vi "h5_init_2D_config.vi"(7 "scan_config":T1={"v0 name"="radiant (nm)", "v0 num"=808, "v1 name"="none", "v1 num"=808, "scan_values"=[], "num rows"=808, "measurement"=0, "v0_config"={"hardware"=enum."radiant (nm)", "options"="", "repeats"=4, "loops"=1, "VISA"="COM9", "override_VISA"=TRUE}, "v1_config"={"hardware"=enum."radiant (nm)", "options"="", "repeats"=4, "loops"=1, "VISA"="COM9", "override_VISA"=TRUE}, "scope_config"={"VISA"="lecroy", "channels"=[enum."Channel 1"], "timeout (ms)"=100000, "max_points"=2500, "averages"=50, "noise filter"=enum."None"}} {"scope_config"."averages" min=1; "scope_config"."max_points" items=["50"=50, "100"=100, "250"=250, "500"=500, "1000"=1000, "2500"=2500, "5K"=5000, "10K"=10000, "25K"=25000, "50K"=50000, "100K"=100000, "250K"=250000, "500K"=500000, "1M"=1000000, "2M"=2000000, "2.5M"=2500000, "5M"=5000000, "10M"=10000000, "25M"=25000000, "50M"=50000000, "100M"=100000000]; "v1_config"."loops" min=1; "v1_config"."repeats" min=1; "v0_config"."loops" min=1; "v0_config"."repeats" min=1}) -> (15 "error out":errorcluster)   [LabVIEW 2017, in "tools.lvlib"]
uses:
  tools.lvlib
  <vilib>/UPVI/lvhdf5/attribute.llb/Simple H5Awrite.xnode
  <vilib>/UPVI/lvhdf5/attribute.llb/LVH5A Operation.ctl
  <vilib>/UPVI/lvhdf5/library.llb/HDF5 Ref.ctl
  <vilib>/UPVI/lvhdf5/attribute.llb/Simple H5Awrite (Variant).vi
  <vilib>/UPVI/lvhdf5/attribute.llb/Cluster to Attribute Array.xnode
  <vilib>/Utility/VariantDataType/GetClusterInfo.vi
  <vilib>/Utility/VariantDataType/VariantType.lvlib
  <vilib>/Utility/VariantDataType/GetTypeInfo.vi
  ctrl/var_list.ctl
  core/var_config.ctl
  hardware/lecroy/scope_config.ctl
  hardware/lecroy/lecroy.lvlib
  core/scan_config.ctl
panel:
  in  "scan_config 2":T1={"v0 name"="radiant (nm)", "v0 num"=808, "v1 name"="none", "v1 num"=808, "scan_values"=[], "num rows"=808, "measurement"=0, "v0_config"={"hardware"=enum."radiant (nm)", "options"="", "repeats"=4, "loops"=1, "VISA"="COM9", "override_VISA"=TRUE}, "v1_config"={"hardware"=enum."radiant (nm)", "options"="", "repeats"=4, "loops"=1, "VISA"="COM9", "override_VISA"=TRUE}, "scope_config"={"VISA"="lecroy", "channels"=[enum."Channel 1"], "timeout (ms)"=100000, "max_points"=2500, "averages"=50, "noise filter"=enum."None"}} {"scope_config"."averages" min=1; "scope_config"."max_points" items=["50"=50, "100"=100, "250"=250, "500"=500, "1000"=1000, "2500"=2500, "5K"=5000, "10K"=10000, "25K"=25000, "50K"=50000, "100K"=100000, "250K"=250000, "500K"=500000, "1M"=1000000, "2M"=2000000, "2.5M"=2500000, "5M"=5000000, "10M"=10000000, "25M"=25000000, "50M"=50000000, "100M"=100000000]; "v1_config"."loops" min=1; "v1_config"."repeats" min=1; "v0_config"."loops" min=1; "v0_config"."repeats" min=1}
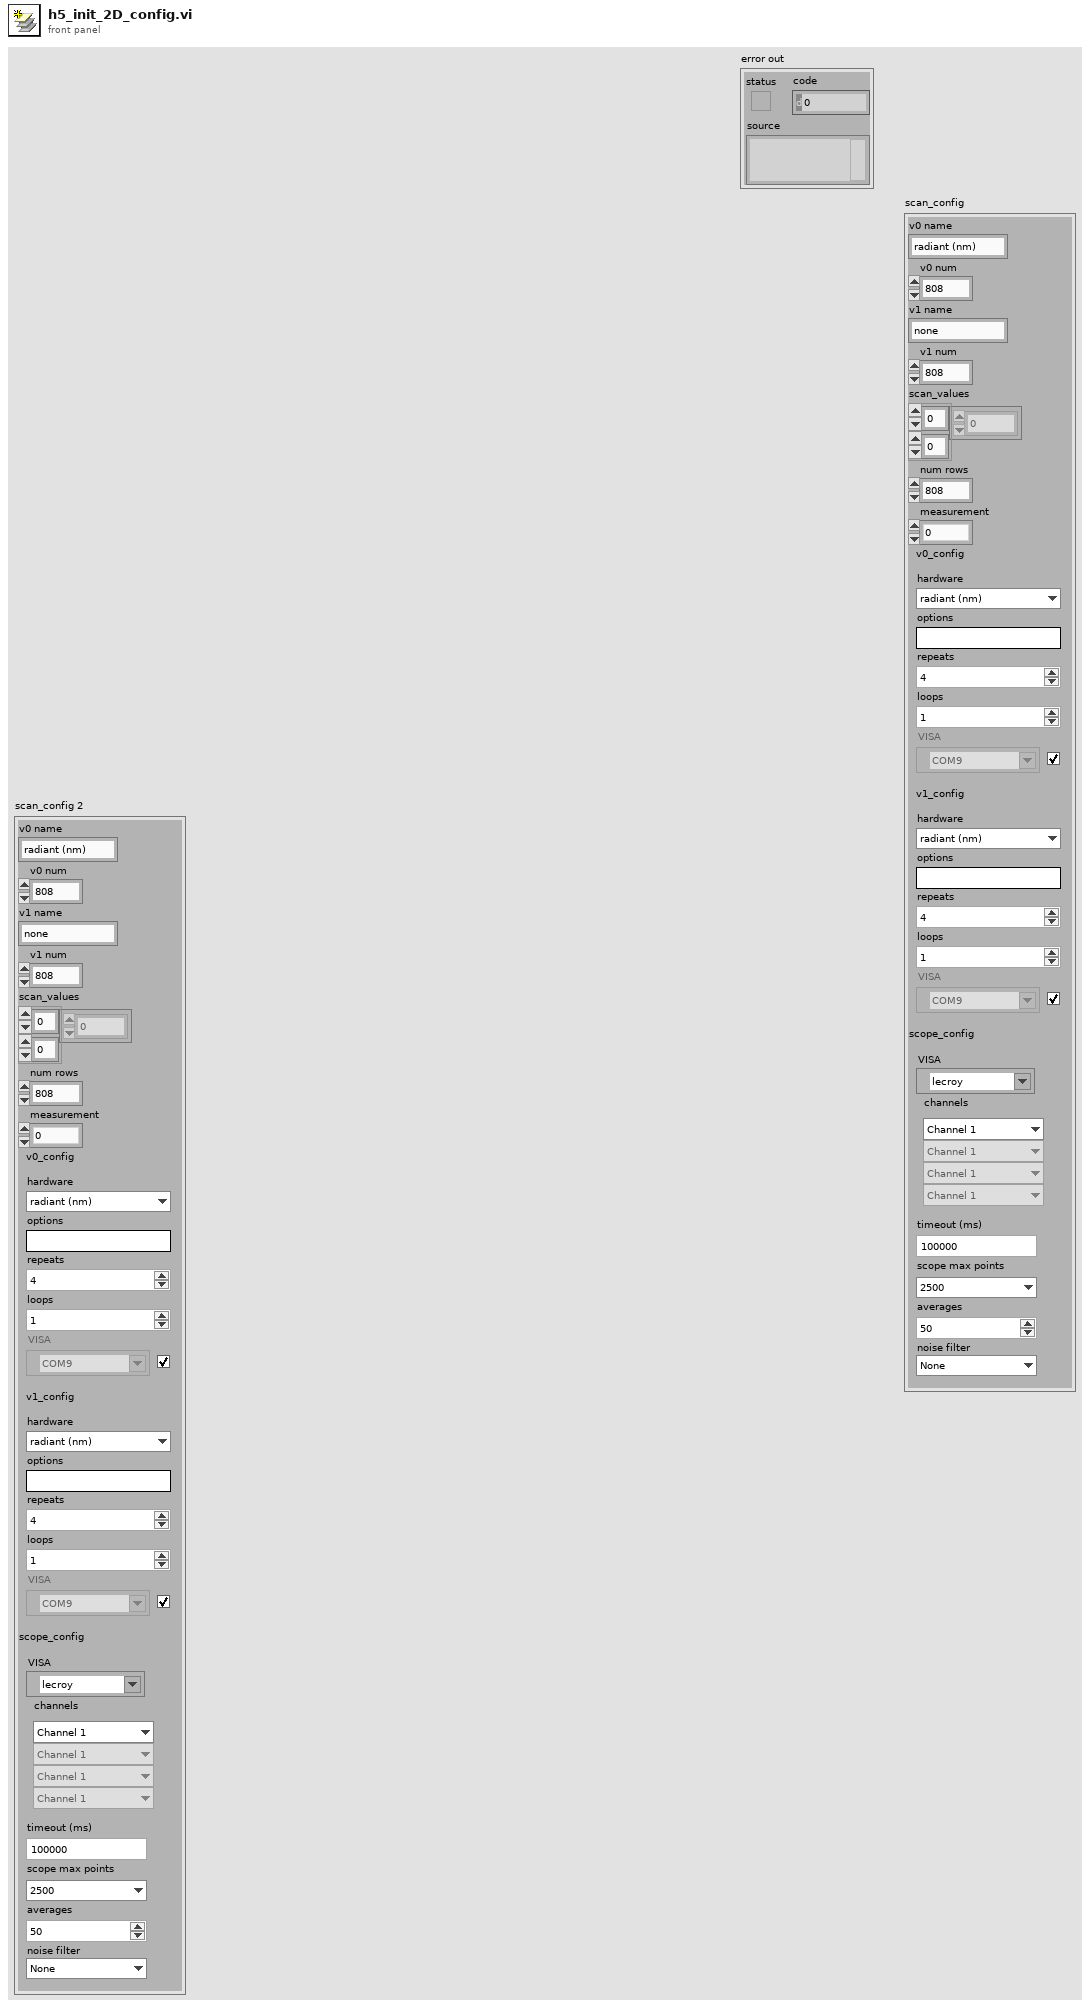
[diagram p1: front panel]
types:
  T1 = typedef "tools.lvlib/scan_config.ctl" = cluster{"v0 name":string, "v0 num":i32, "v1 name":string, "v1 num":i32, "scan_values":dbl[][], "num rows":i32, "measurement":i32, "v0_config":T2, "v1_config":T2, "scope_config":T4}
  T2 = typedef "tools.lvlib/var_config.ctl" = cluster{"hardware":T3, "options":string, "repeats":i32, "loops":i32, "VISA":refnum<visa-resource-name>, "override_VISA":bool}
  T3 = typedef "var_list.ctl" = enum16{"none", "AO voltage (V)", "delay (s)", "generic", "microwaves (GHz)", "radiant (nm)", "radiant thg (nm)", "sirah (nm)", "sirah_shg (nm)", "tenma voltage (V)", "wait (s)", "wf_freq (Hz)", "wf_amp (V)", "wf_amp_multi (V)", "wf_offset (V)", "wf_low_level (V)", "wf_high_level (V)", "wf_period (s)", "wf_pulse_width (s)", "wf_sample_rate (Sa/s)", "wf_multi_amp", "wf_multi_freq", "wf_arb_4chan", "WS7 setpoint (nm)"}
  T4 = typedef "lecroy.lvlib/scope_config.ctl" = cluster{"VISA":refnum<visa-resource-name>, "channels":enum16{"Channel 1", "Channel 2", "Channel 3", "Channel 4"}[], "timeout (ms)":u32, "max_points":i32, "averages":i32, "noise filter":enum16{"None", "+0.5 bit", "+1 bit", "+1.5 bits", "+2 bits", "+2.5 bits", "+3 bits"}}
  T5 = cluster{"num rows":i32, "v0_config":T2, "v1_config":T2, "scope_config":T4}
  T6 = typedef "HDF5 Ref.ctl" = refnum<k1>
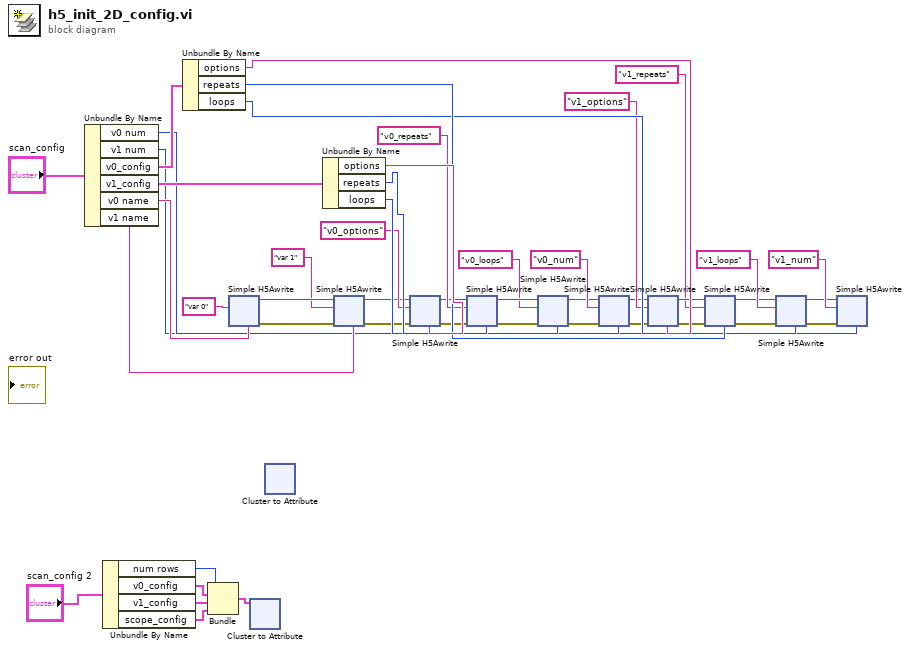
[diagram p0: block diagram]
diagram:
  n1 = Unbundle By Name("scan_config") -> ("v0 num"=w36:i32, "v1 num"=w35:i32, "v0_config"=w40:T2, "v1_config"=w39:T2, "v0 name"=w38:string, "v1 name"=w37:string)
  n2 = Unbundle By Name("scan_config 2") -> ("num rows"=w1:i32, "v0_config"=w5:T2, "v1_config"=w4:T2, "scope_config"=w3:T4)
  n3 = Unbundle By Name(w40) -> ("options"=w46:string, "repeats"=w43:i32, "loops"=w42:i32)
  n4 = Bundle("num rows"=w1, "v0_config"=w5, "v1_config"=w4, "scope_config"=w3) -> (w2:T5)  [unwired: 1 in]
  n5 = xnode "Simple H5Awrite"("Name"="var 0", "Value"=w38) -> ("HDF5 Ref out"=w31:T6, "error out"=w32:errorcluster)  [unwired: 3 in]
  n6 = xnode "Cluster to Attribute"("Cluster"=w2) -> ()  [unwired: 5 in, 3 out]
  n7 = xnode "Cluster to Attribute"() -> ()  [unwired: 6 in, 3 out]
  n8 = Unbundle By Name(w39) -> ("options"=w47:string, "repeats"=w45:i32, "loops"=w44:i32)
  n9 = xnode "Simple H5Awrite"("HDF5 Ref"=w31, "Name"="var 1", "error in (no error)"=w32, "Value"=w37) -> ("HDF5 Ref out"=w30:T6, "error out"=w29:errorcluster)  [unwired: 1 in]
  n10 = xnode "Simple H5Awrite"("HDF5 Ref"=w30, "Name"="v0_options", "error in (no error)"=w29, "Value"=w47) -> ("HDF5 Ref out"=w26:T6, "error out"=w25:errorcluster)  [unwired: 1 in]
  n11 = xnode "Simple H5Awrite"("HDF5 Ref"=w26, "Name"="v0_repeats", "error in (no error)"=w25, "Value"=w45) -> ("HDF5 Ref out"=w23:T6, "error out"=w24:errorcluster)  [unwired: 1 in]
  n12 = xnode "Simple H5Awrite"("HDF5 Ref"=w23, "Name"="v0_loops", "error in (no error)"=w24, "Value"=w44) -> ("HDF5 Ref out"=w11:T6, "error out"=w12:errorcluster)  [unwired: 1 in]
  n13 = xnode "Simple H5Awrite"("HDF5 Ref"=w11, "Name"="v0_num", "error in (no error)"=w12, "Value"=w36) -> ("HDF5 Ref out"=w9:T6, "error out"=w10:errorcluster)  [unwired: 1 in]
  n14 = xnode "Simple H5Awrite"("HDF5 Ref"=w9, "Name"="v1_options", "error in (no error)"=w10, "Value"=w46) -> ("HDF5 Ref out"=w20:T6, "error out"=w21:errorcluster)  [unwired: 1 in]
  n15 = xnode "Simple H5Awrite"("HDF5 Ref"=w20, "Name"="v1_repeats", "error in (no error)"=w21, "Value"=w43) -> ("HDF5 Ref out"=w15:T6, "error out"=w16:errorcluster)  [unwired: 1 in]
  n16 = xnode "Simple H5Awrite"("HDF5 Ref"=w15, "Name"="v1_loops", "error in (no error)"=w16, "Value"=w42) -> ("HDF5 Ref out"=w8:T6, "error out"=w7:errorcluster)  [unwired: 1 in]
  n17 = xnode "Simple H5Awrite"("HDF5 Ref"=w8, "Name"="v1_num" ("v1_num"), "error in (no error)"=w7, "Value"=w35) -> ()  [unwired: 1 in, 2 out]
